vi "_Update Cal or Res Data.vi"(4 "error in (no error)":errorcluster, 6 "Table Type":T1) -> (0 "error out":errorcluster)   [LabVIEW 2015]
uses:
  Type/_Table Type.ctl
  _RT Global.vi
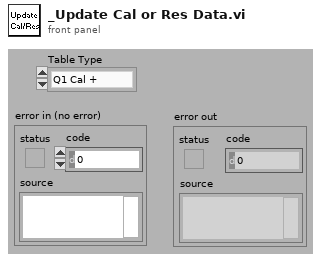
[diagram p1: front panel]
types:
  T1 = typedef "_Table Type.ctl" = enum8{"Q1 Cal +", "Q2 Cal +", "Q1 Cal -", "Q2 Cal -", "Q1 Res Hi +", "Q2 Res Hi +", "Q1 Res Med +", "Q2 Res Med +", "Q1 Res Lo +", "Q2 Res Lo +", "Q1 Res Hi -", "Q2 Res Hi -", "Q1 Res Med -", "Q2 Res Med -", "Q1 Res Lo -", "Q2 Res Lo -"}
  T2 = typedef "Semaphore RefNum" = refnum<k1>
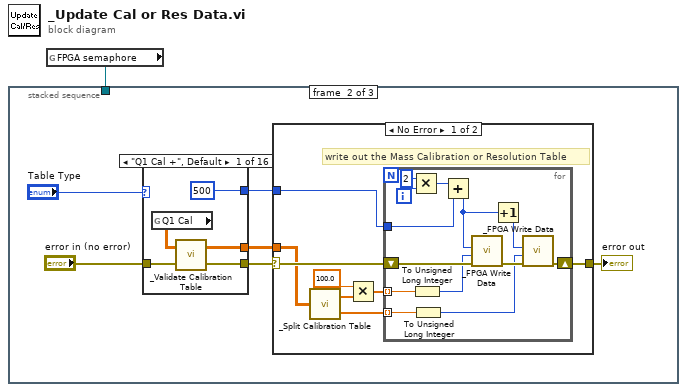
[diagram p0: block diagram]
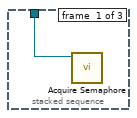
[diagram p2: hidden frame]
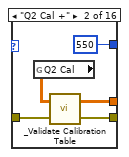
[diagram p3: hidden frame]
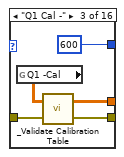
[diagram p4: hidden frame]
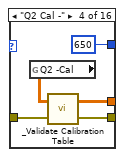
[diagram p5: hidden frame]
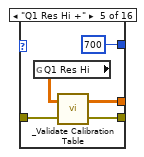
[diagram p6: hidden frame]
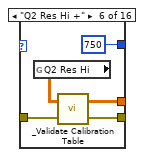
[diagram p7: hidden frame]
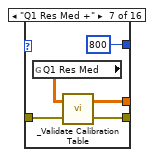
[diagram p8: hidden frame]
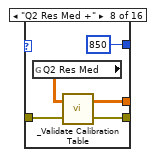
[diagram p9: hidden frame]
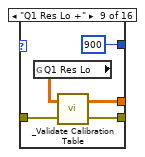
[diagram p10: hidden frame]
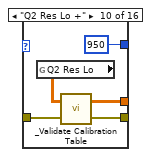
[diagram p11: hidden frame]
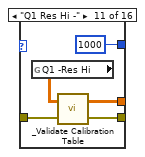
[diagram p12: hidden frame]
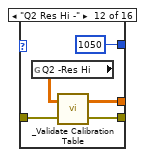
[diagram p13: hidden frame]
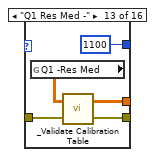
[diagram p14: hidden frame]
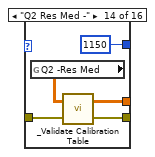
[diagram p15: hidden frame]
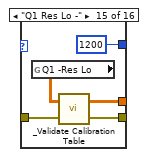
[diagram p16: hidden frame]
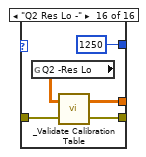
[diagram p17: hidden frame]
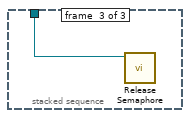
[diagram p19: hidden frame]
diagram:
  n1 = global read "_RT Global.vi" "FPGA semaphore"() -> (w1:T2)
  n2 = stacked-sequence {
    tunnel: w1 -> [w2 _ w111]
    frame #0 {
      n3 = call <vilib>:"Acquire Semaphore.vi"("semaphore"=w2) -> ()  [unwired: 2 in, 5 out]
    }
    frame #1 {
      n4 = case shown="\"Q1 Cal +\", Default" "Table Type" {
        tunnel: [w11 w15 w21 w25 w30 w35 w40 w45 w50 w55 w60 w65 w70 w75 w80 w85] -> w3
        tunnel: [500 ("y") 550 ("y") 600 ("y") 650 ("y") 700 ("y") 750 ("y") 800 ("y") 850 ("y") 900 ("y") 950 ("y") 1000 ("y") 1050 ("y") 1100 ("y") 1150 ("y") 1200 ("y") 1250 ("y")] -> w4
        tunnel: "error in (no error)" -> [w10 w16 w20 w26 w31 w36 w41 w46 w51 w56 w61 w66 w71 w76 w81 w86]
        tunnel: [w9 w14 w19 w24 w29 w34 w39 w44 w49 w54 w59 w64 w69 w74 w79 w84] -> w5
        frame "Q1 Cal +", Default {
          n5 = global read "_RT Global.vi" "Q1 Cal"() -> (w12:dbl[][])
          n6 = call "_Validate Calibration Table.vi"("error in (no error)"=w10, "Calibration In"=w12) -> ("error out"=w9:errorcluster, "Calibration Out"=w11:dbl[][])
        }
        frame "Q2 Cal +" {
          n7 = global read "_RT Global.vi" "Q2 Cal"() -> (w17:dbl[][])
          n8 = call "_Validate Calibration Table.vi"("error in (no error)"=w16, "Calibration In"=w17) -> ("error out"=w14:errorcluster, "Calibration Out"=w15:dbl[][])
        }
        frame "Q1 Cal -" {
          n9 = global read "_RT Global.vi" "Q1 -Cal"() -> (w22:dbl[][])
          n10 = call "_Validate Calibration Table.vi"("error in (no error)"=w20, "Calibration In"=w22) -> ("error out"=w19:errorcluster, "Calibration Out"=w21:dbl[][])
        }
        frame "Q2 Cal -" {
          n11 = global read "_RT Global.vi" "Q2 -Cal"() -> (w27:dbl[][])
          n12 = call "_Validate Calibration Table.vi"("error in (no error)"=w26, "Calibration In"=w27) -> ("error out"=w24:errorcluster, "Calibration Out"=w25:dbl[][])
        }
        frame "Q1 Res Hi +" {
          n13 = global read "_RT Global.vi" "Q1 Res Hi"() -> (w32:dbl[][])
          n14 = call "_Validate Calibration Table.vi"("error in (no error)"=w31, "Calibration In"=w32) -> ("error out"=w29:errorcluster, "Calibration Out"=w30:dbl[][])
        }
        frame "Q2 Res Hi +" {
          n15 = global read "_RT Global.vi" "Q2 Res Hi"() -> (w37:dbl[][])
          n16 = call "_Validate Calibration Table.vi"("error in (no error)"=w36, "Calibration In"=w37) -> ("error out"=w34:errorcluster, "Calibration Out"=w35:dbl[][])
        }
        frame "Q1 Res Med +" {
          n17 = global read "_RT Global.vi" "Q1 Res Med"() -> (w42:dbl[][])
          n18 = call "_Validate Calibration Table.vi"("error in (no error)"=w41, "Calibration In"=w42) -> ("error out"=w39:errorcluster, "Calibration Out"=w40:dbl[][])
        }
        frame "Q2 Res Med +" {
          n19 = global read "_RT Global.vi" "Q2 Res Med"() -> (w47:dbl[][])
          n20 = call "_Validate Calibration Table.vi"("error in (no error)"=w46, "Calibration In"=w47) -> ("error out"=w44:errorcluster, "Calibration Out"=w45:dbl[][])
        }
        frame "Q1 Res Lo +" {
          n21 = global read "_RT Global.vi" "Q1 Res Lo"() -> (w52:dbl[][])
          n22 = call "_Validate Calibration Table.vi"("error in (no error)"=w51, "Calibration In"=w52) -> ("error out"=w49:errorcluster, "Calibration Out"=w50:dbl[][])
        }
        frame "Q2 Res Lo +" {
          n23 = global read "_RT Global.vi" "Q2 Res Lo"() -> (w57:dbl[][])
          n24 = call "_Validate Calibration Table.vi"("error in (no error)"=w56, "Calibration In"=w57) -> ("error out"=w54:errorcluster, "Calibration Out"=w55:dbl[][])
        }
        frame "Q1 Res Hi -" {
          n25 = global read "_RT Global.vi" "Q1 -Res Hi"() -> (w62:dbl[][])
          n26 = call "_Validate Calibration Table.vi"("error in (no error)"=w61, "Calibration In"=w62) -> ("error out"=w59:errorcluster, "Calibration Out"=w60:dbl[][])
        }
        frame "Q2 Res Hi -" {
          n27 = global read "_RT Global.vi" "Q2 -Res Hi"() -> (w67:dbl[][])
          n28 = call "_Validate Calibration Table.vi"("error in (no error)"=w66, "Calibration In"=w67) -> ("error out"=w64:errorcluster, "Calibration Out"=w65:dbl[][])
        }
        frame "Q1 Res Med -" {
          n29 = global read "_RT Global.vi" "Q1 -Res Med"() -> (w72:dbl[][])
          n30 = call "_Validate Calibration Table.vi"("error in (no error)"=w71, "Calibration In"=w72) -> ("error out"=w69:errorcluster, "Calibration Out"=w70:dbl[][])
        }
        frame "Q2 Res Med -" {
          n31 = global read "_RT Global.vi" "Q2 -Res Med"() -> (w77:dbl[][])
          n32 = call "_Validate Calibration Table.vi"("error in (no error)"=w76, "Calibration In"=w77) -> ("error out"=w74:errorcluster, "Calibration Out"=w75:dbl[][])
        }
        frame "Q1 Res Lo -" {
          n33 = global read "_RT Global.vi" "Q1 -Res Lo"() -> (w82:dbl[][])
          n34 = call "_Validate Calibration Table.vi"("error in (no error)"=w81, "Calibration In"=w82) -> ("error out"=w79:errorcluster, "Calibration Out"=w80:dbl[][])
        }
        frame "Q2 Res Lo -" {
          n35 = global read "_RT Global.vi" "Q2 -Res Lo"() -> (w87:dbl[][])
          n36 = call "_Validate Calibration Table.vi"("error in (no error)"=w86, "Calibration In"=w87) -> ("error out"=w84:errorcluster, "Calibration Out"=w85:dbl[][])
        }
      }
      n37 = case shown="No Error" w5 {
        selector: w5 -> [w91 w110]
        tunnel: [w92 w110] -> w8
        tunnel: w4 -> [w90 _]
        tunnel: w3 -> [w89 _]
        frame No Error {
          # "write out the Mass Calibration or Resolution Table"
          n38 = call "_Split Calibration Table.vi"("Calibration"=w89) -> ("Mass"=w96:dbl[], "DAC"=w95:dbl[])
          n39 = Multiply(x=100.0, y=w96) -> (x*y=w94:dbl[])
          n40 = for {
            shift-right: [w98] -> w92
            shift-left: w91 -> [w109]
            tunnel: w94 -> [w108] mode=indexing
            tunnel: w95 -> [w107] mode=indexing
            tunnel: w90 -> [w101]
            i -> [w106]
            n41 = Multiply(x=2, y=w106) -> (x*y=w104:i32)
            n42 = To Unsigned Long Integer(number=w108) -> (unsigned 32bit integer=w100:u32)
            n43 = To Unsigned Long Integer(number=w107) -> (unsigned 32bit integer=w99:u32)
            n44 = Add(x=w104, y=w101) -> (x+y=w97:i32)
            n45 = call "_FPGA Write Data.vi"("error in"=w109, "Data"=w100, "Address"=w97) -> ("error out"=w103:errorcluster)  [unwired: 3 in, 2 out]
            n46 = Increment(x=w97) -> (x+1=w102:i32)
            n47 = call "_FPGA Write Data.vi"("error in"=w103, "Data"=w99, "Address"=w102) -> ("error out"=w98:errorcluster)  [unwired: 3 in, 2 out]
          }
        }
        frame Error {
        }
      }
      "error out" <- w8
    }
    frame #2 {
      n48 = call <vilib>:"Release Semaphore.vi"("semaphore"=w111) -> ()  [unwired: 1 in, 6 out]
    }
  }
